vi "MT Apply Pulse Shaping Filter (MSK).vi"(0 "symbols":dbl[](array[numeric]) min=0.0 max=127.0 format="%.2f", 5 "pulse shaping filter coefficients":dbl[](array[numeric]) format="%.2f", 7 "samples per symbol (16)":i32=16, 9 "symbol rate (Hz)":dbl=1.0, 11 "error in (no error)":errorcluster, 13 "reset? (T)":bool=TRUE) -> (4 "output complex waveform":T1={"t0"=0.0, "dt"=1.0, "Y"=[]} {"Y" format="%.3f"; "dt" format="%^.2e"; "t0" format="%.4f"}, 15 "error out":errorcluster)   [LabVIEW 2020, in "niDMT.lvlib"]
doc: "This polymorphic instance applies a pulse-shaping filter to an input stream comprised of MSK- or CPM-modulated symbols. The VI performs filtering using the specified <B>pulse shaping filter coefficients</B> followed by accumulation on the phase of the information symbols to generate the oversampled MSK- or CPM-modulated complex baseband waveform. This process is the digital equivalent of continuous-time analog frequency modulation."
uses:
  <vilib>/addons/Modulation/niDMT.lvlib
  <vilib>/addons/Modulation/Analog/controls/Complex Data Waveform.ctl
  <vilib>/addons/Modulation/niAMT.lvlib
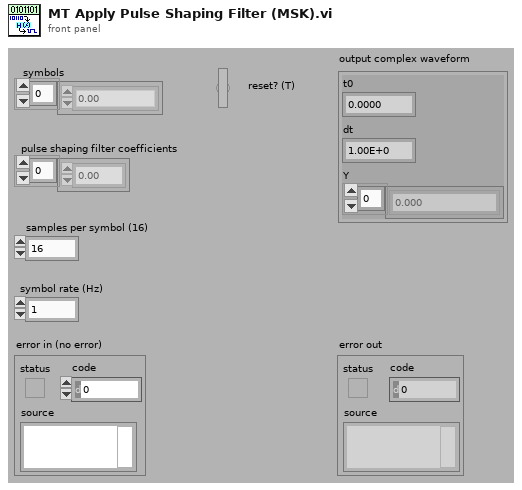
[diagram p1: front panel]
types:
  T1 = typedef "niAMT.lvlib/Complex Data Waveform.ctl" = cluster{"t0":dbl, "dt":dbl, "Y":cdb[]}
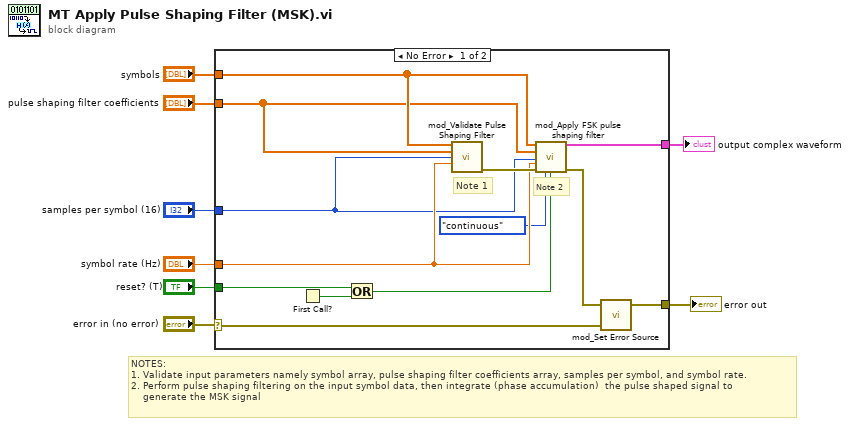
[diagram p0: block diagram]
diagram:
  # "NOTES:\n1. Validate input parameters namely symbol array, pulse shaping filter coefficients array, samples per symbol, and symbol rate.\n2. Perform pulse shaping filtering on the input symbol data, then integrate (phase accumulation)  the pulse shaped signal to \n    generate the MSK signal"
  n1 = case shown="No Error" "error in (no error)" {
    selector: "error in (no error)" -> [w13 w22]
    tunnel: "symbols" -> [w16 _]
    tunnel: "pulse shaping filter coefficients" -> [w15 _]
    tunnel: "symbol rate (Hz)" -> [w14 _]
    tunnel: [w21 _] -> w4
    tunnel: [w11 w22] -> w3
    tunnel: "reset? (T)" -> [w20 _]
    tunnel: "samples per symbol (16)" -> [w10 _]
    frame No Error {
      # "Note 2"
      # "Note 1"
      n2 = First Call?() -> (First Call?: T/F=w19:bool)
      n3 = Or(x=w20, y=w19) -> (x .or. y?=w18:bool)
      n4 = call <vilib>:"mod_Validate Pulse Shaping Filter.vi"("symbols"=w16, "pulse shaping filter coefficients"=w15, "samples per symbol (16)"=w10, "symbol Rate, Hz"=w14) -> ("error out"=w17:errorcluster)  [unwired: 11 out]
      n5 = call <vilib>:"mod_Apply FSK pulse shaping filter.vi"("symbols"=w16, "pulse shaping filter coefficients"=w15, "samples per symbol (16)"=w10, "symbol rate"=w14, "error in (no error)"=w17, "symbol phase continuity"=enum16{"continuous", "discontinuous"}."continuous", "reset? (T)"=w18) -> ("output complex waveform"=w21:T1, "error out"=w12:errorcluster)  [unwired: 7 out]
      n6 = call <vilib>:"mod_Set Error Source.vi"("initial error in (no error)"=w13, "final error in (no error)"=w12) -> ("error out"=w11:errorcluster)  [unwired: 3 out]
    }
    frame Error {
    }
  }
  "output complex waveform" <- w4
  "error out" <- w3
